vi "Register for IOLink broadcast.vi"(8 "error in":errorcluster) -> (0 "error out":errorcluster)   [LabVIEW 2024, in "Hardware Controller.lvlib"]
doc: "registers the helper loops for the io link module broadcasts\n\n_____\nCreated using DQMH Event Scripter 7.0.0.1280."
uses:
  Hardware Controller.lvlib
  Register for IOLink broadcast Argument--cluster.ctl
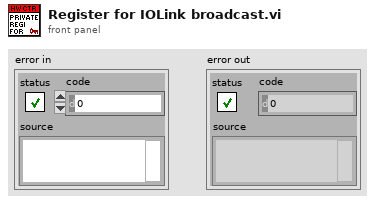
[diagram p1: front panel]
types:
  T1 = typedef "Hardware Controller.lvlib/Register for IOLink broadcast Argument--cluster.ctl" = cluster{"Boolean":bool}
  T2 = typedef "Hardware Controller.lvlib/Request Events--cluster.ctl" = cluster{"Stop Module":refnum<user-event>, "Show Panel":refnum<user-event>, "Hide Panel":refnum<user-event>, "Get Module Execution Status":refnum<user-event>, "Show Diagram":refnum<user-event>, "Private":cluster{"Start System State Broadcast Helper Loop":refnum<user-event>, "Launch EtherCat":refnum<user-event>, "Register for Broadcast EtherCAT system state":refnum<user-event>, "Launch IOLink":refnum<user-event>, "Register for IOLink broadcast":refnum<user-event>}, "Launch all Hardware":refnum<user-event>, "Write I16":refnum<user-event>, "Write U16":refnum<user-event>, "Start EtherCAT Conection":refnum<user-event>, "Ready Drive":refnum<user-event>, "Clear System Fault":refnum<user-event>, "Close EtherCAT Connection":refnum<user-event>}
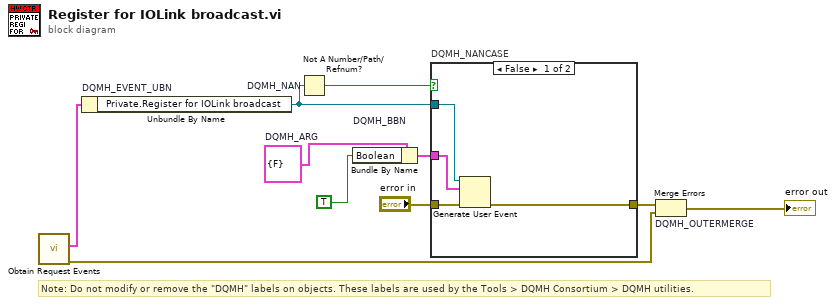
[diagram p0: block diagram]
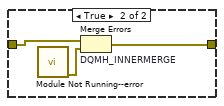
[diagram p2: hidden frame]
diagram:
  w4 = T1 {"Boolean"=FALSE}  # DQMH_ARG
  # "Note: Do not modify or remove the \"DQMH\" labels on objects. These labels are used by the Tools > DQMH Consortium > DQMH utilities."
  n1 = call "Obtain Request Events.vi"() -> ("error out"=w2:errorcluster, "Hardware Controller Request Events"=w1:T2)  [unwired: 10 in]
  n2 = Unbundle By Name "DQMH_EVENT_UBN"(w1) -> ("Private.Register for IOLink broadcast"=w6:refnum<user-event>)
  n3 = Not A Number/Path/Refnum? "DQMH_NAN"(number/path/refnum=w6) -> (NaN/Path/Refnum?=w7:bool)
  n4 = Bundle By Name "DQMH_BBN"(cluster=w4, "Boolean"=TRUE) -> (w8:T1)
  n5 = case "DQMH_NANCASE" shown="False" w7 {
    tunnel: "error in" -> [w14 w17]
    tunnel: [w13 w16] -> w5
    tunnel: w6 -> [w12 _]
    tunnel: w8 -> [w11 _]
    frame False {
      n6 = Generate User Event(user event=w12, event data cluster=w11, error in=w14) -> (error out=w13:errorcluster)  [unwired: 1 in, 1 out]
    }
    frame True {
      n7 = call "Module Not Running--error.vi"() -> ("error out"=w15:errorcluster)  [unwired: 11 in]
      n8 = Merge Errors "DQMH_INNERMERGE"(w17, w15) -> (w16:errorcluster)
    }
  }
  n9 = Merge Errors "DQMH_OUTERMERGE"(w5, w2) -> (→"error out":errorcluster)
